vi "WPs and Obstacles 5.vi"() -> (0 "Obstacle Real Lats and Longs":cluster{"Obs Lats":dbl[], "Obs Longs":dbl[]} {"Obs Longs" format="%#_8g"; "Obs Lats" format="%#_8g"}, 1 "WP Real Lats and Longs":cluster{"WP Lats":dbl[], "WP Longs":dbl[]} {"WP Longs" format="%#_8g"; "WP Lats" format="%#_8g"}, 2 "Sim Matrx":u8[][](array[numeric]), 3 "Real WP Map":T1(graph), 5 "Sim Course":picture)   [LabVIEW 2014]
panel:
  in  "Obstacle Real Longs":dbl[](array[numeric])=[81.2678, 81.267312, 81.267112, 81.267332, 81.267916, 81.267137, 81.267874, 81.267301, 81.267913, 81.26772] format="%#_8g"
  in  "Obstacle Real Lats":dbl[](array[numeric])=[37.1524, 37.152256, 37.152877, 37.152903, 37.152565, 37.152792, 37.152806, 37.152779, 37.152868, 37.152484] format="%#_8g"
  in  "WP Real Longs":dbl[](array[numeric])=[81.2671, 81.26711, 81.267112, 81.267332, 81.267916, 81.267137, 81.267874, 81.267301, 81.267913, 81.26772] format="%#_8g"
  in  "WP Real Lats":dbl[](array[numeric])=[37.1528, 37.15281, 37.152877, 37.152903, 37.152565, 37.152792, 37.152806, 37.152779, 37.152868, 37.152484] format="%#_8g"
  # "Waypoint and Obstacles 5 (Uses Paint)"
  # "Added Global sim painted map"
  # "Inputs:"
  # "Sim Lats and Longs not being used"
  # "20"
  # "12"
  # "Outputs:"
  # "Sim Painted Picture to matrix"
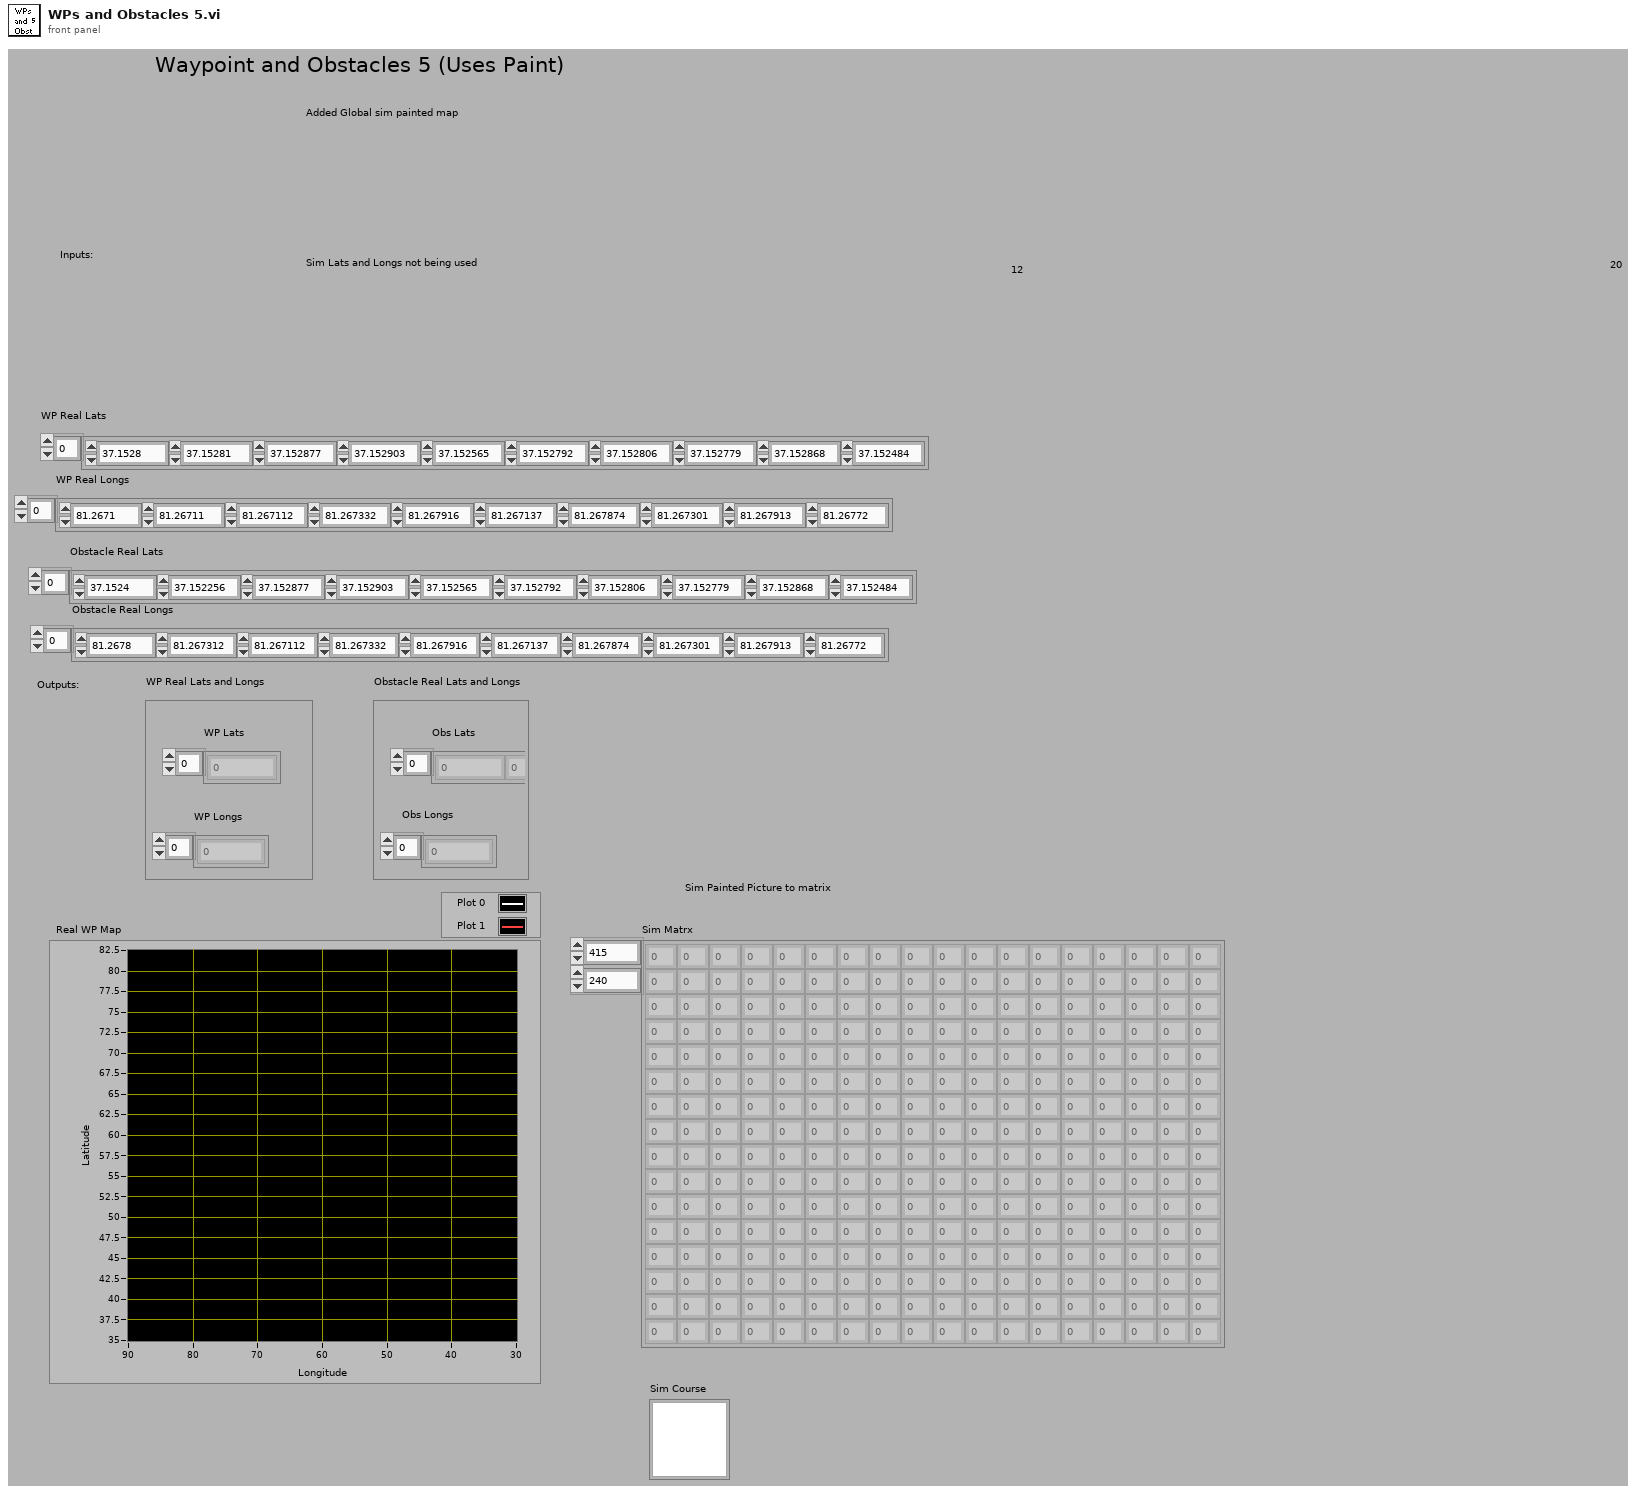
[diagram p1: front panel]
types:
  T1 = cluster{"Obstacle Longs":dbl[], "Obstacle Lats":dbl[]}[]
  T2 = cluster{"Obstacle Real Lats":dbl[], "Obstacle Real Longs":dbl[]}
  T3 = cluster{"WP Real Lats":dbl[], "WP Real Longs":dbl[]}
  T4 = cluster{"Obstacle Longs":dbl[], "Obstacle Lats":dbl[]}
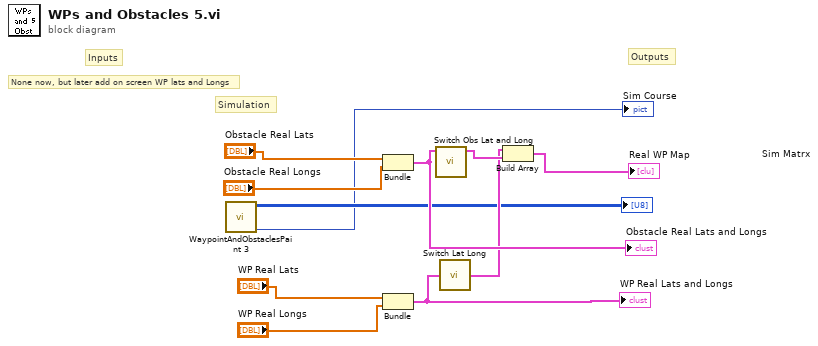
[diagram p0: block diagram]
diagram:
  # "None now, but later add on screen WP lats and Longs"
  # "Simulation"
  # "Inputs"
  # "Outputs"
  n1 = call "WaypointAndObstaclesPaint 3.vi"() -> ("Sim Course"=→"Sim Course":picture, 3:→"Sim Matrx":u8[][])  [unwired: 10 in]
  n2 = Bundle("Obstacle Real Lats"="Obstacle Real Lats", "Obstacle Real Longs"="Obstacle Real Longs") -> (w10:T2)  [unwired: 1 in]
  "Obstacle Real Lats and Longs" <- w10
  n3 = Bundle("WP Real Lats"="WP Real Lats", "WP Real Longs"="WP Real Longs") -> (w11:T3)  [unwired: 1 in]
  "WP Real Lats and Longs" <- w11
  n4 = call "Switch Obs Lat and Long.vi"("Obstacle Lats and Longs for GIC"=w10) -> ("Obstacle Lats and Longs switched"=w9:T4)  [unwired: 10 in]
  n5 = call "Switch Lat Long.vi"("WP Lats and Longs for GIC"=w11) -> ("WP Lats and Longs switched"=w8:cluster{"WP Longs":dbl[], "WP Lats":dbl[]})
  n6 = Build Array(w8, w9) -> (→"Real WP Map":T1)
